vi "Run_VI_Named_specific.vi"(8 "Run VI Named String":string, 11 "Multi Run Row":T1 {"Row Duration (mins)" format="%#.1f"; "Row No" min=0; "Trace Gas Concentration (%)" min=0.0 format="%#.2f"; "Emission Rate (l/min)" format="%#.2f"; "Tunnel Speed" format="%#.2f"; "Start X" format="%#.2f"; "Start Y" format="%#.2f"; "Start Z" format="%#.2f"; "End X" format="%#.2f"; "End Y" format="%#.2f"; "End Z" format="%#.2f"; "Averaging time (min)" min=0.0 format="%#.1f"}) -> (0 "Scalable Time (Sec)":dbl format="%.2f", 1 "Fixed Time (Sec)":dbl format="%.2f", 2 "Channel Names":string[](array[string]), 3 "Checks":string[](array[string]), 4 "Error String":string, 5 "Check Meas Setup?":bool, 6 "Check for start NaNs?":bool)   [LabVIEW 2010]
uses:
  Gen Trav/Traverse_cluster.ctl
  Gen Trav/Spacing.ctl
  Controls/Multi_run_mode.ctl
  Globals/Preference_global.vi
panel:
  # "X           Y            Z"
  # "Start"
  # "End"
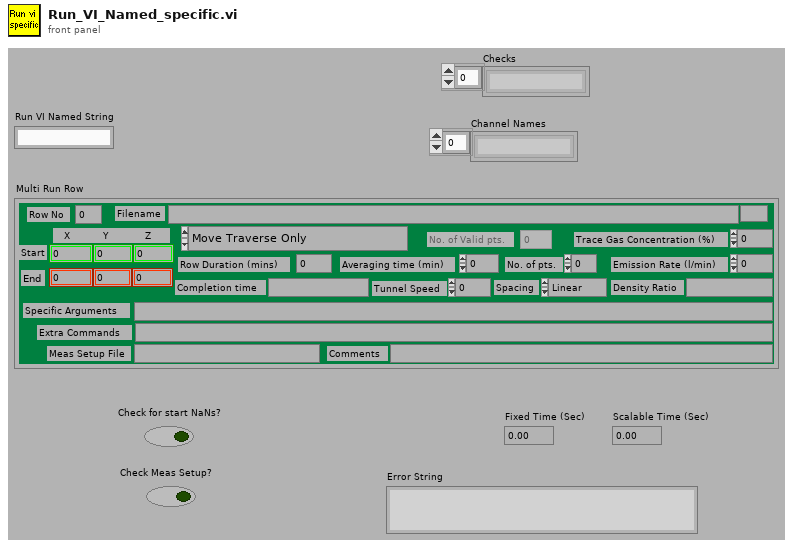
[diagram p1: front panel]
types:
  T1 = typedef "Traverse_cluster.ctl" = cluster{"Start X":dbl, "Start Y":dbl, "Start Z":dbl, "End X":dbl, "End Y":dbl, "End Z":dbl, "No. of pts.":i32, "Spacing":T2, "Filename":path, "Tunnel Speed":dbl, "Averaging time (min)":dbl, "Extra Commands":string, "Specific Arguments":string, "Emission Rate (l/min)":dbl, "Trace Gas Concentration (%)":dbl, "Density Ratio":string, "Comments":string, "Row No":i32, "Row Type Selector":T3, "Completion time":string, "Row Duration (mins)":dbl, "No. of Valid pts.":i32, "Meas Setup File":string}
  T2 = typedef "Spacing.ctl" = enum16{"Linear", "Log", "Gauss", "Specified", "N/A"}
  T3 = typedef "Multi_run_mode.ctl" = enum16{"Move Traverse Only", "Set Tunnel Speed Only", "Set Source Only", "Set Measurement Conditions", "Single Measurement", "Vertical Profile", "Lateral Profile", "Longitudinal Profile", "Explore Volume", "Multi-Axis Profile", "Auto Calibrate", "Meas Fast FID Bkgnd", "Check Beam Power", "Scanning Valve Measurement", "Run VI Named:", "Set ADAM Ch", "Wait (minutes)", "Send Message", "Synchronize With:", "Fall Back to this Row", "Turn Off Row Repeating", "Blank Row"}
  T4 = typedef "Beam_Type.ctl" = u16
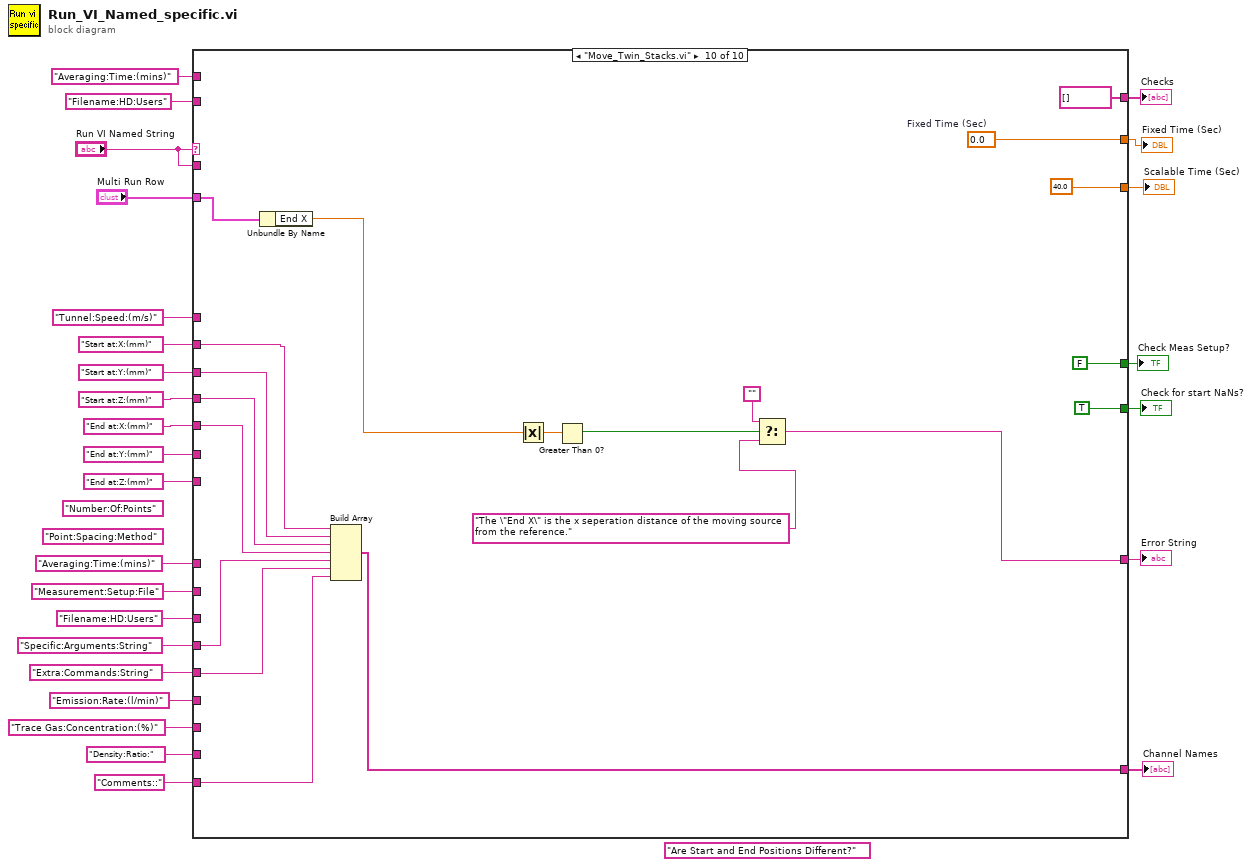
[diagram p0: block diagram]
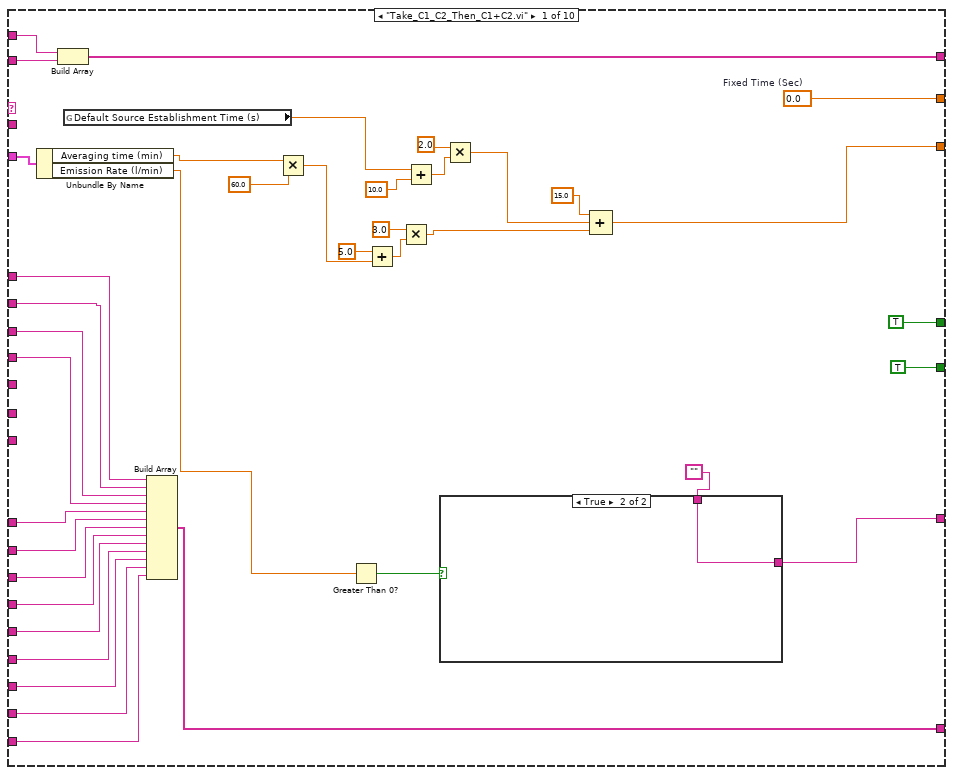
[diagram p2: hidden frame]
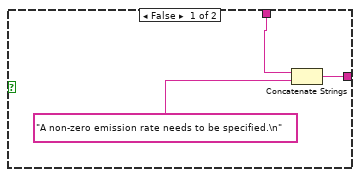
[diagram p3: hidden frame]
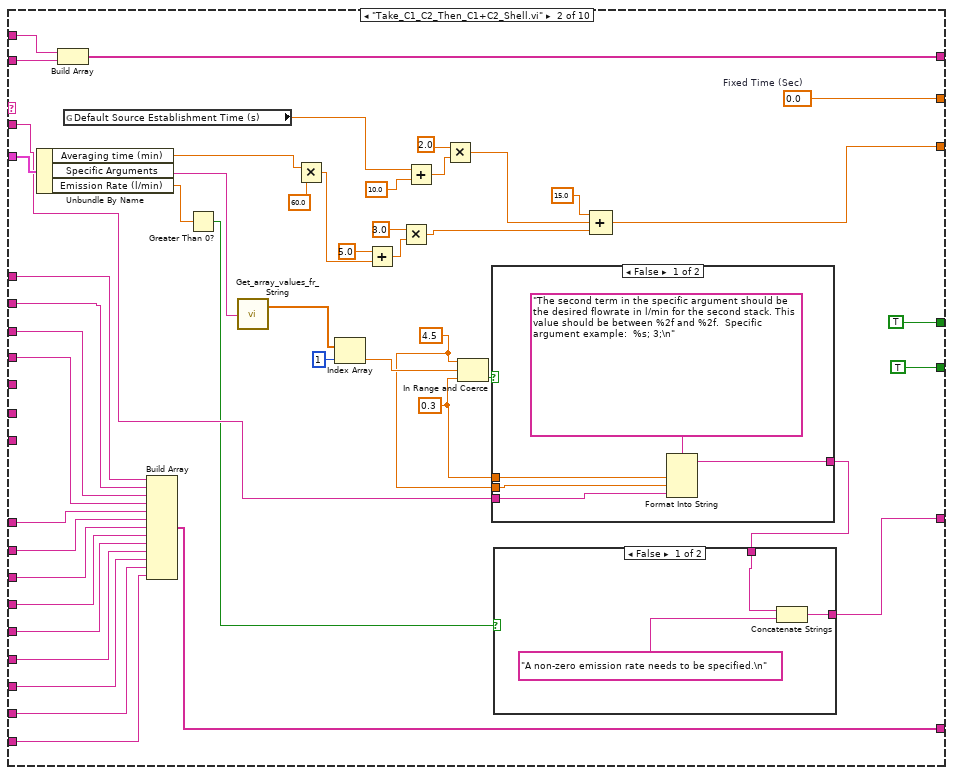
[diagram p4: hidden frame]
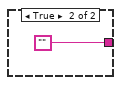
[diagram p6: hidden frame]
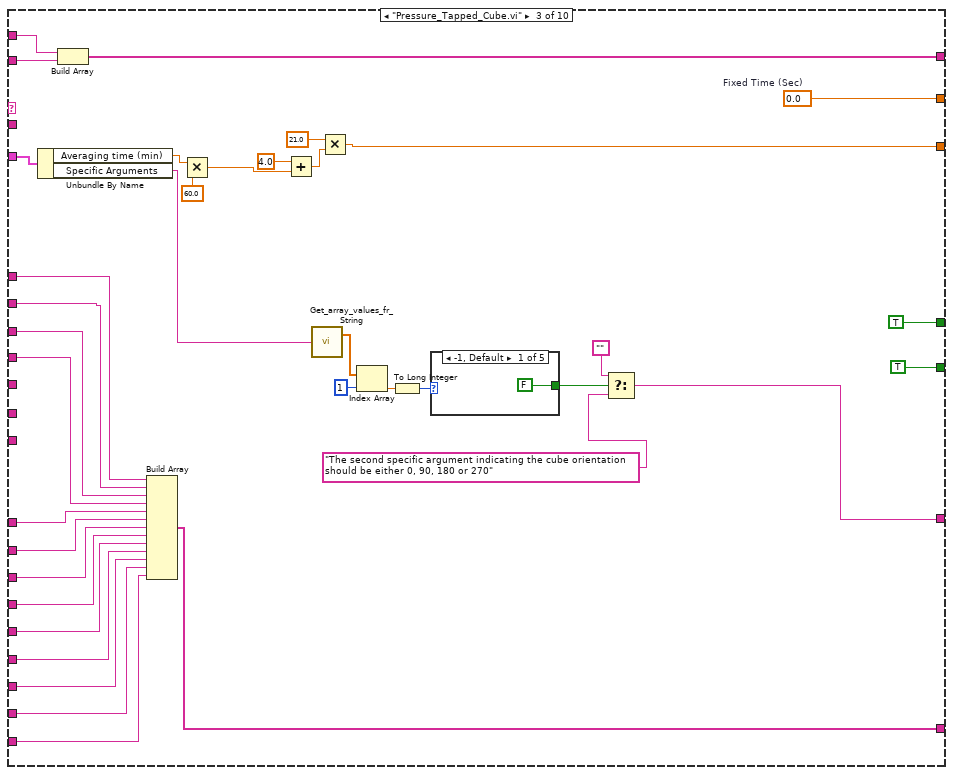
[diagram p7: hidden frame]
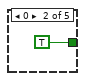
[diagram p8: hidden frame]
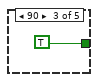
[diagram p9: hidden frame]
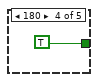
[diagram p10: hidden frame]
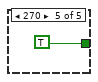
[diagram p11: hidden frame]
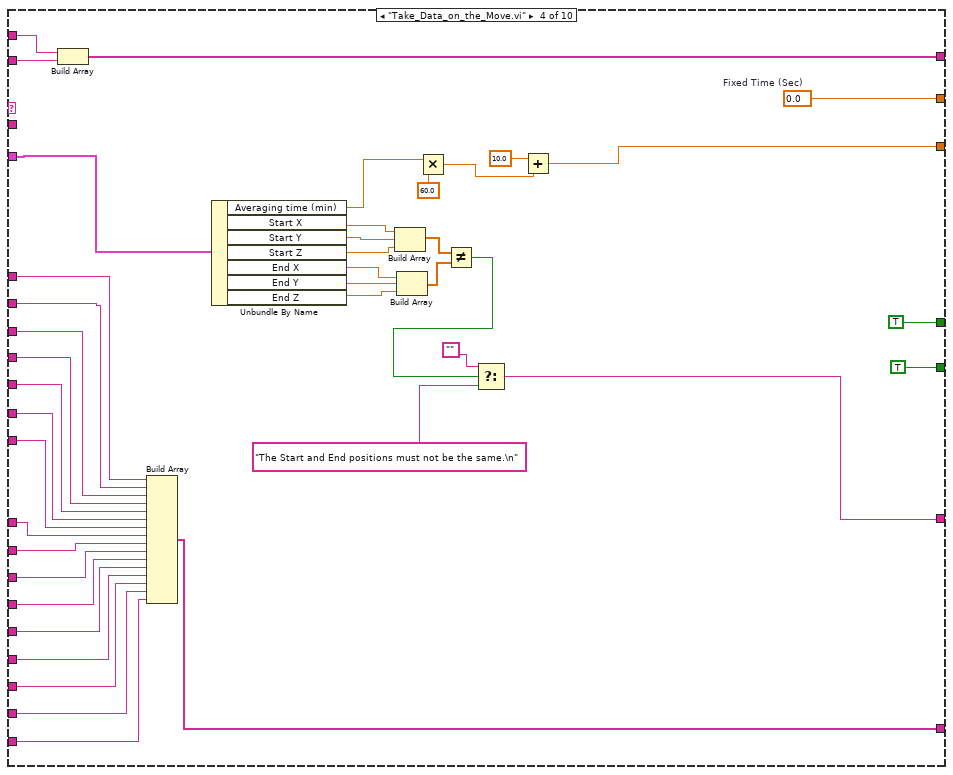
[diagram p12: hidden frame]
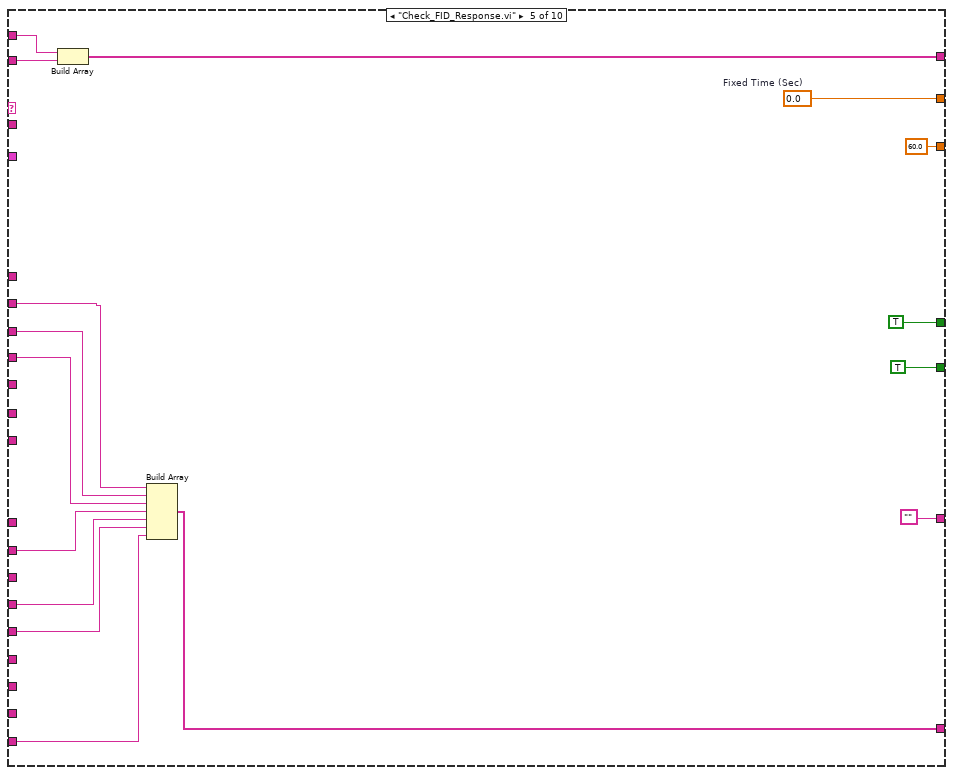
[diagram p13: hidden frame]
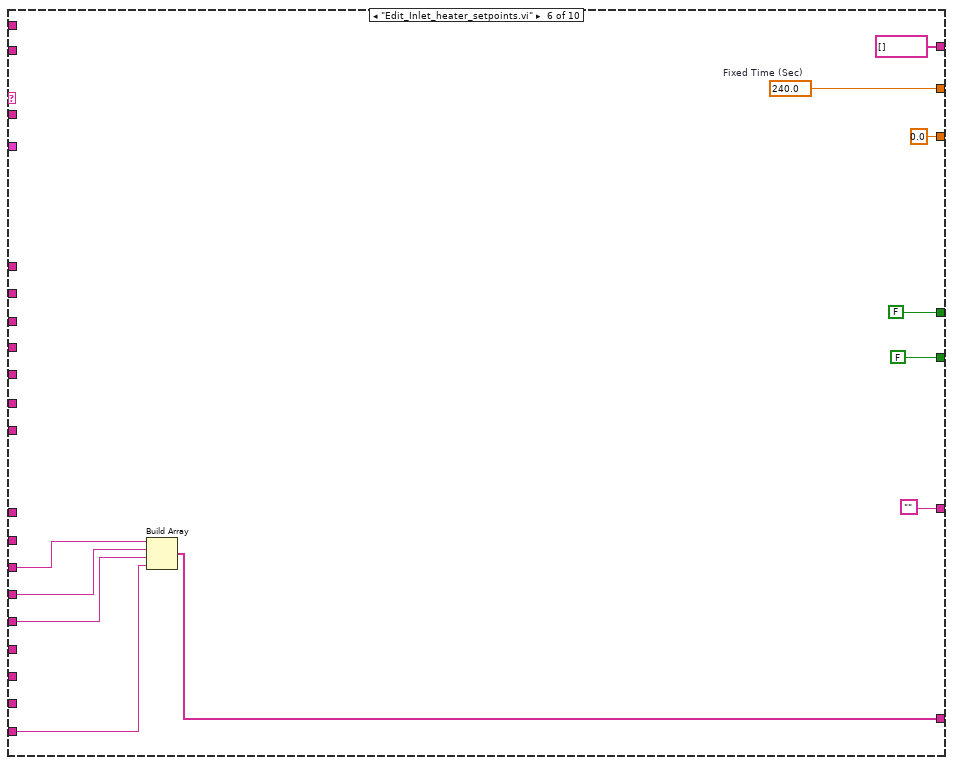
[diagram p14: hidden frame]
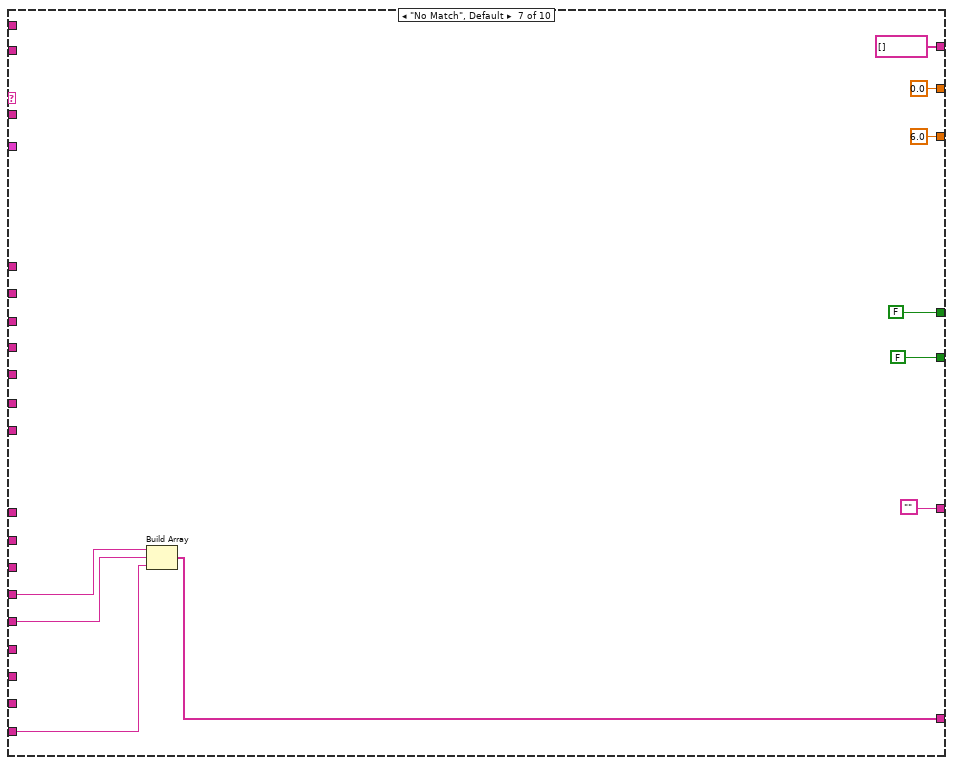
[diagram p15: hidden frame]
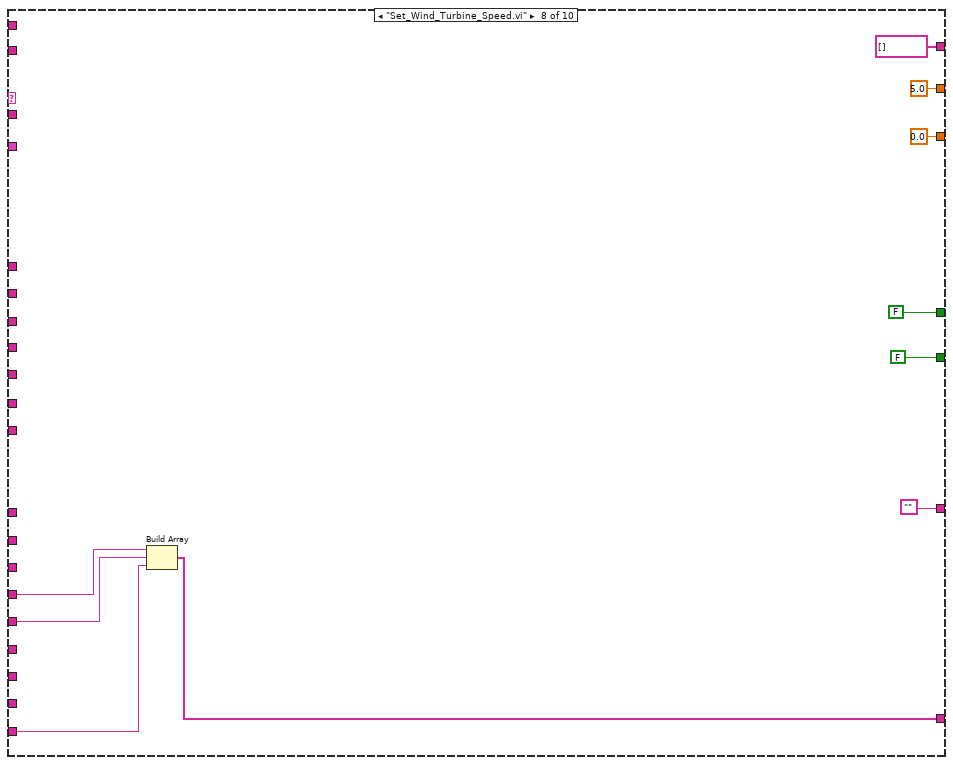
[diagram p16: hidden frame]
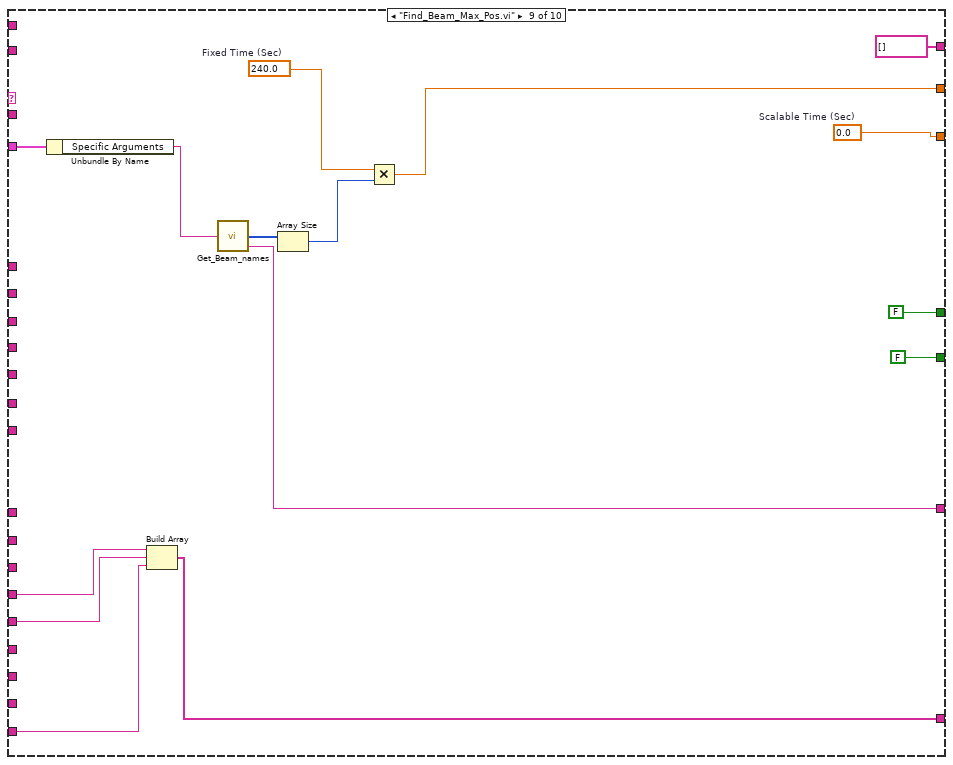
[diagram p17: hidden frame]
diagram:
  (unwired) "Point:Spacing:Method" ("Label for value")
  (unwired) "Number:Of:Points" ("Label for value")
  (unwired) "Are Start and End Positions Different?" ("Label for value")
  n1 = case shown="\"Move_Twin_Stacks.vi\"" "Run VI Named String" {
    tunnel: "Multi Run Row" -> [w66 w117 w164 w176 _ _ _ _ w265 w292]
    tunnel: [w65 w116 w163 w210 w226 w237 0.0 ("Fixed Time (Sec)") 5.0 ("Fixed Time (Sec)") w259 w291] -> w26
    tunnel: [w51 w102 w137 w174 60.0 ("value") 0.0 ("value") 6.0 ("value") 0.0 ("value") w260 40.0 ("value")] -> w25
    tunnel: "Averaging:Time:(mins)" ("Label for value") -> [w50 w101 w160 w208 w225 _ _ _ _ _]
    tunnel: "Filename:HD:Users" ("Label for value") -> [w49 w100 w159 w207 w224 _ _ _ _ _]
    tunnel: [TRUE TRUE TRUE TRUE TRUE FALSE FALSE FALSE FALSE TRUE] -> w22
    tunnel: [TRUE TRUE TRUE TRUE TRUE FALSE FALSE FALSE FALSE FALSE] -> w21
    tunnel: [w46 w97 w156 w204 w221 string[] [] string[] [] string[] [] string[] [] string[] []] -> w20
    tunnel: "Tunnel:Speed:(m/s)" ("Label for value") -> [w45 w96 w155 w203 _ _ _ _ _ _]
    tunnel: "Start at:X:(mm)" ("Label for value") -> [w44 w95 w154 w202 w220 _ _ _ _ w288]
    tunnel: "Start at:Y:(mm)" ("Label for value") -> [w43 w94 w153 w201 w219 _ _ _ _ w287]
    tunnel: "Start at:Z:(mm)" ("Label for value") -> [w42 w93 w152 w200 w218 _ _ _ _ w286]
    tunnel: "Averaging:Time:(mins)" ("Label for value") -> [w41 w92 w151 w199 _ _ _ _ _ _]
    tunnel: "Measurement:Setup:File" ("Label for value") -> [w40 w91 w150 w198 w217 _ _ _ _ _]
    tunnel: "Filename:HD:Users" ("Label for value") -> [w39 w90 w149 w197 _ w227 _ _ _ _]
    tunnel: "Specific:Arguments:String" ("Label for value") -> [w38 w89 w148 w196 w216 w234 w245 w255 w270 w274]
    tunnel: "Extra:Commands:String" ("Label for value") -> [w37 w88 w147 w195 w215 w233 w244 w254 w269 w273]
    tunnel: "Emission:Rate:(l/min)" ("Label for value") -> [w36 w87 w146 w194 _ _ _ _ _ _]
    tunnel: "Trace Gas:Concentration:(%)" ("Label for value") -> [w35 w86 w145 w193 _ _ _ _ _ _]
    tunnel: "Density:Ratio:" ("Label for value") -> [w34 w85 w144 w192 _ _ _ _ _ _]
    tunnel: "Comments::" ("Label for value") -> [w33 w84 w143 w191 w214 w232 w243 w253 w268 w282]
    tunnel: [w32 w83 w142 w190 w213 w231 w242 w252 w267 w285] -> w6
    tunnel: [w30 w71 w128 w173 "" "" "" "" w258 w276] -> w5
    tunnel: "End at:X:(mm)" ("Label for value") -> [_ _ _ w172 _ _ _ _ _ w283]
    tunnel: "End at:Y:(mm)" ("Label for value") -> [_ _ _ w171 _ _ _ _ _ _]
    tunnel: "End at:Z:(mm)" ("Label for value") -> [_ _ _ w170 _ _ _ _ _ _]
    tunnel: "Run VI Named String" -> [_ w77 _ _ _ _ _ _ _ _]
    frame "Take_C1_C2_Then_C1+C2.vi" {
      w65 = 0.0  # Fixed Time (Sec)
      n2 = Unbundle By Name(w66) -> ("Averaging time (min)"=w54:dbl, "Emission Rate (l/min)"=w29:dbl)
      n3 = Build Array(w50, w49) -> (w46:string[])
      n4 = global read "Preference_global.vi" "Default Source Establishment Time (s)"() -> (w55:dbl)
      n5 = Build Array(w45, w44, w43, w42, w41, w40, w39, w38, w37, w36, w35, w34, w33) -> (w32:string[])
      n6 = Multiply(x=w54, y=60.0) -> (x*y=w52:dbl)
      n7 = Greater Than 0?(x=w29) -> (x > 0?=w28:bool)
      n8 = Add(x=5.0, y=w52) -> (x+y=w58:dbl)
      n9 = Multiply(x=3.0, y=w58) -> (x*y=w62:dbl)
      n10 = Add(x=w55, y=10.0) -> (x+y=w60:dbl)
      n11 = case shown="True" w28 {
        tunnel: "" -> [w68 w70]
        tunnel: [w67 w70] -> w30
        frame False {
          n12 = Concatenate Strings(w68, "A non-zero emission rate needs to be specified.\n") -> (w67:string)
        }
        frame True {
        }
      }
      n13 = Multiply(x=2.0, y=w60) -> (x*y=w63:dbl)
      n14 = Compound Arithmetic op=ADD(15.0 ("value"), w63, w62) -> (w51:dbl)
    }
    frame "Take_C1_C2_Then_C1+C2_Shell.vi" {
      w75 = 4.5 ("upper limit")
      w76 = 0.3 ("lower limit")
      w116 = 0.0  # Fixed Time (Sec)
      n15 = Unbundle By Name(w117) -> ("Averaging time (min)"=w105:dbl, "Specific Arguments"=w80:string, "Emission Rate (l/min)"=w74:dbl)
      n16 = Build Array(w101, w100) -> (w97:string[])
      n17 = global read "Preference_global.vi" "Default Source Establishment Time (s)"() -> (w106:dbl)
      n18 = Build Array(w96, w95, w94, w93, w92, w91, w90, w89, w88, w87, w86, w85, w84) -> (w83:string[])
      n19 = Greater Than 0?(x=w74) -> (x > 0?=w73:bool)
      n20 = call "Get_array_values_fr_String.vi"("String Value"=w80) -> ("Numeric Array"=w82:dbl[])  [unwired: 1 out]
      n21 = Multiply(x=w105, y=60.0) -> (x*y=w103:dbl)
      n22 = Index Array(array=w82, index=1) -> (element=w79:dbl)
      n23 = Add(x=5.0, y=w103) -> (x+y=w109:dbl)
      n24 = Multiply(x=3.0, y=w109) -> (x*y=w113:dbl)
      n25 = Add(x=w106, y=10.0) -> (x+y=w111:dbl)
      n26 = Multiply(x=2.0, y=w111) -> (x*y=w114:dbl)
      n27 = In Range and Coerce(upper limit=w75, x=w79, lower limit=w76) -> (In Range?=w78:bool)  [unwired: 1 out]
      n28 = case shown="False" w78 {
        tunnel: [w122 ""] -> w72
        tunnel: w77 -> [w126 _]
        tunnel: w76 -> [w125 _]
        tunnel: w75 -> [w124 _]
        frame False {
          n29 = Format Into String(format string="The second term in the specific argument should be the desired flowrate in l/min for the second stack. This value should be between %2f and %2f.  Specific argument example:  %s; 3;\n", w125, w124, w126) -> (resulting string=w122:string)  [unwired: 2 in, 1 out]
        }
        frame True {
        }
      }
      n30 = case shown="False" w73 {
        tunnel: w72 -> [w119 w121]
        tunnel: [w118 w121] -> w71
        frame False {
          n31 = Concatenate Strings(w119, "A non-zero emission rate needs to be specified.\n") -> (w118:string)
        }
        frame True {
        }
      }
      n32 = Compound Arithmetic op=ADD(15.0 ("value"), w114, w113) -> (w102:dbl)
    }
    frame "Pressure_Tapped_Cube.vi" {
      w163 = 0.0  # Fixed Time (Sec)
      n33 = Unbundle By Name(w164) -> ("Averaging time (min)"=w162:dbl, "Specific Arguments"=w129:string)
      n34 = Build Array(w160, w159) -> (w156:string[])
      n35 = Build Array(w155, w154, w153, w152, w151, w150, w149, w148, w147, w146, w145, w144, w143) -> (w142:string[])
      n36 = Multiply(x=w162, y=60.0) -> (x*y=w138:dbl)
      n37 = Add(x=4.0, y=w138) -> (x+y=w141:dbl)
      n38 = call "Get_array_values_fr_String.vi"("String Value"=w129) -> ("Numeric Array"=w131:dbl[])  [unwired: 1 out]
      n39 = Multiply(x=21.0, y=w141) -> (x*y=w137:dbl)
      n40 = Index Array(array=w131, index=1) -> (element=w132:dbl)
      n41 = To Long Integer(number=w132) -> (32bit integer=w133:i32)
      n42 = case shown="-1, Default" w133 {
        tunnel: [FALSE TRUE TRUE TRUE TRUE] -> w136
        frame -1, Default {
        }
        frame 0 {
        }
        frame 90 {
        }
        frame 180 {
        }
        frame 270 {
        }
      }
      n43 = Select(t="", s=w136, f="The second specific argument indicating the cube orientation should be either 0, 90, 180 or 270") -> (s? t:f=w128:string)
    }
    frame "Take_Data_on_the_Move.vi" {
      w210 = 0.0  # Fixed Time (Sec)
      n44 = Build Array(w208, w207) -> (w204:string[])
      n45 = Build Array(w203, w202, w201, w200, w172, w171, w170, w199, w198, w197, w196, w195, w194, w193, w192, w191) -> (w190:string[])
      n46 = Unbundle By Name(w176) -> ("Averaging time (min)"=w175:dbl, "Start X"=w177:dbl, "Start Y"=w178:dbl, "Start Z"=w179:dbl, "End X"=w180:dbl, "End Y"=w181:dbl, "End Z"=w182:dbl)
      n47 = Build Array(w177, w178, w179) -> (w184:dbl[])
      n48 = Build Array(w180, w181, w182) -> (w183:dbl[])
      n49 = Multiply(x=w175, y=60.0) -> (x*y=w188:dbl)
      n50 = Not Equal?(x=w184, y=w183) -> (x != y?=w187:bool)
      n51 = Select(t="", s=w187, f="The Start and End positions must not be the same.\n" ("Format String")) -> (s? t:f=w173:string)
      n52 = Add(x=10.0, y=w188) -> (x+y=w174:dbl)
    }
    frame "Check_FID_Response.vi" {
      w226 = 0.0  # Fixed Time (Sec)
      n53 = Build Array(w225, w224) -> (w221:string[])
      n54 = Build Array(w220, w219, w218, w217, w216, w215, w214) -> (w213:string[])
    }
    frame "Edit_Inlet_heater_setpoints.vi" {
      w237 = 240.0  # Fixed Time (Sec)
      n55 = Build Array(w227, w234, w233, w232) -> (w231:string[])
    }
    frame "No Match", Default {
      n56 = Build Array(w245, w244, w243) -> (w242:string[])
    }
    frame "Set_Wind_Turbine_Speed.vi" {
      n57 = Build Array(w255, w254, w253) -> (w252:string[])
    }
    frame "Find_Beam_Max_Pos.vi" {
      w264 = 240.0  # Fixed Time (Sec)
      w260 = 0.0  # Scalable Time (Sec)
      n58 = Unbundle By Name(w265) -> ("Specific Arguments"=w261:string)
      n59 = Build Array(w270, w269, w268) -> (w267:string[])
      n60 = call "Get_Beam_names.vi"("String Value"=w261) -> ("Beam Array"=w262:T4[], "Error Comments"=w258:string)  [unwired: 1 out]
      n61 = Array Size(array=w262) -> (size(s)=w263:i32)
      n62 = Multiply(x=w264, y=w263) -> (x*y=w259:dbl)
    }
    frame "Move_Twin_Stacks.vi" {
      w291 = 0.0  # Fixed Time (Sec)
      n63 = Unbundle By Name(w292) -> ("End X"=w279:dbl)
      n64 = Build Array(w288, w287, w286, w283, w274, w273, w282) -> (w285:string[])
      n65 = Absolute Value(x=w279) -> (abs(x)=w278:dbl)
      n66 = Greater Than 0?(x=w278) -> (x > 0?=w281:bool)
      n67 = Select(t="", s=w281, f="The \"End X\" is the x seperation distance of the moving source from the reference.") -> (s? t:f=w276:string)
    }
  }
  "Fixed Time (Sec)" <- w26
  "Scalable Time (Sec)" <- w25
  "Check Meas Setup?" <- w21
  "Error String" <- w5
  "Check for start NaNs?" <- w22
  "Checks" <- w20
  "Channel Names" <- w6
